vi "Skipfire.vi"(8 "error in (no error)":errorcluster, 11 "Node Ptr":T2 format="%.0x") -> (0 "error out":errorcluster)   [LabVIEW 2016, in "DCM System Explorer.lvlib"]
uses:
  DCM System Explorer.lvlib
  <vilib>/NI Veristand/Custom Device API/Custom Device Item Ref.ctl
  <vilib>/Powertrain Controls/Device Drivers/DCM/Skip Fire/RT/Skip Fire Setup.ctl
  Shared/DCM Properties.vi
  <vilib>/NI Veristand/Custom Device API/Get Item Property (String Array).vi
  Shared/DCM Constants and GUIDs.vi
  <vilib>/NI Veristand/Custom Device API/Set Item Property (String Array).vi
  <vilib>/NI VeriStand/Custom Device API/Custom Device API.lvlib
  DCM Shared.lvlib
  <vilib>/Powertrain Controls/Device Drivers/DCM/Skip Fire/RT/DCM - RT - Skip Fire.lvlib
panel:
  in  "_Setup Element":T1 caption="Command Setup"
  in  "_Refresh":bool
  in  "Channel Names":string[](array[string])=["", "", "", "", "", "", "", "", "", "", "", ""]
  in  "Channel Name":string
  in  "_Skipfire Channels":i32[](listbox) caption="Summary"
  in  "_Save Changes?":bool
  in  "Setup":T1[](array[typedef]) caption="Differential I/O Setup"
  in  "Header":cluster{"Section Name":string}={"Section Name"="Skip Fire Setup"}
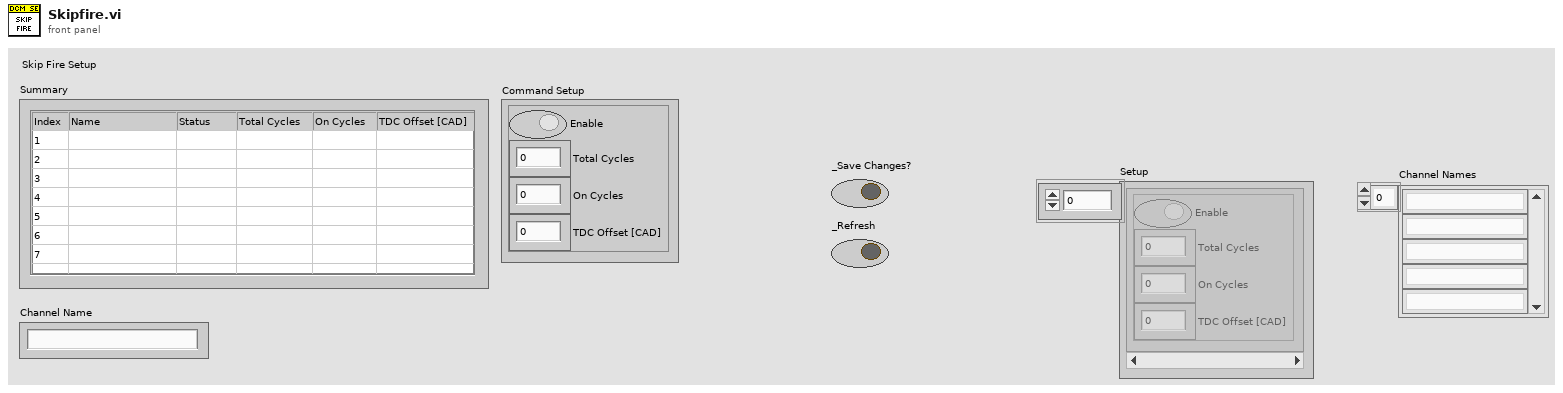
[diagram p1: front panel]
types:
  T1 = typedef "DCM - RT - Skip Fire.lvlib/Skip Fire Setup.ctl" = cluster{"Enable":bool, "Total Cycles":u8, "On Cycles":u8, "TDC Offset [CAD]":sgl}
  T2 = typedef "Custom Device API.lvlib/Custom Device Item Ref.ctl" = u64
  T3 = typedef "Custom Device API.lvlib/Custom Device Commands.ctl" = enum16{"Default", "Item renamed", "Shutdown", "Dynamic button pressed"}
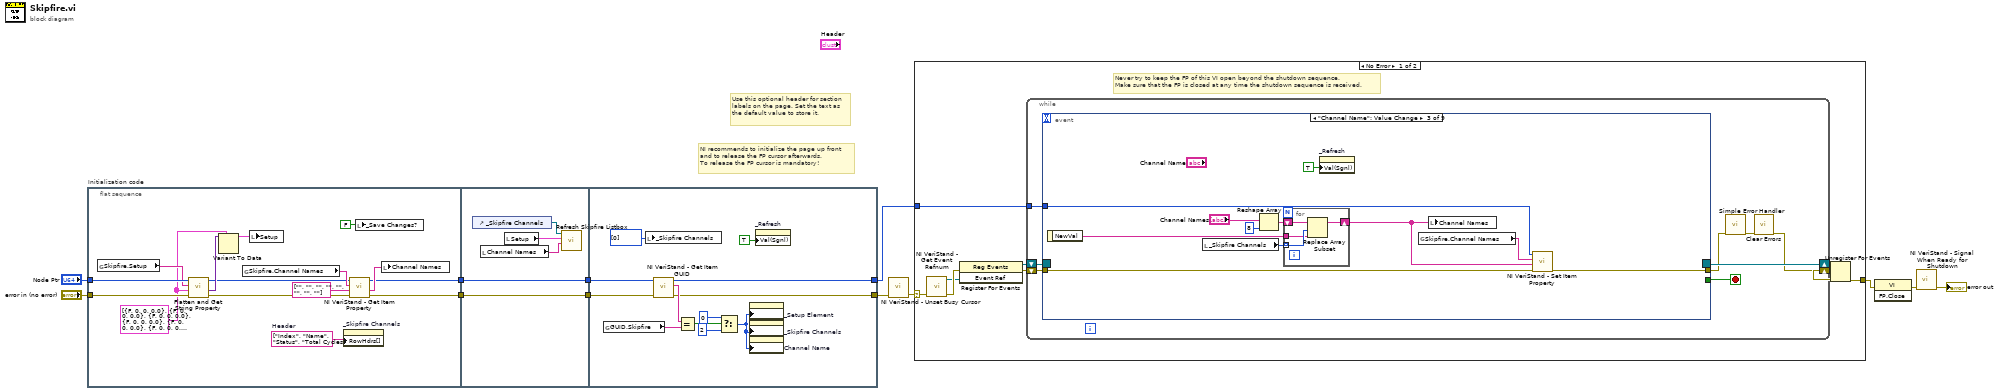
[diagram p0: block diagram]
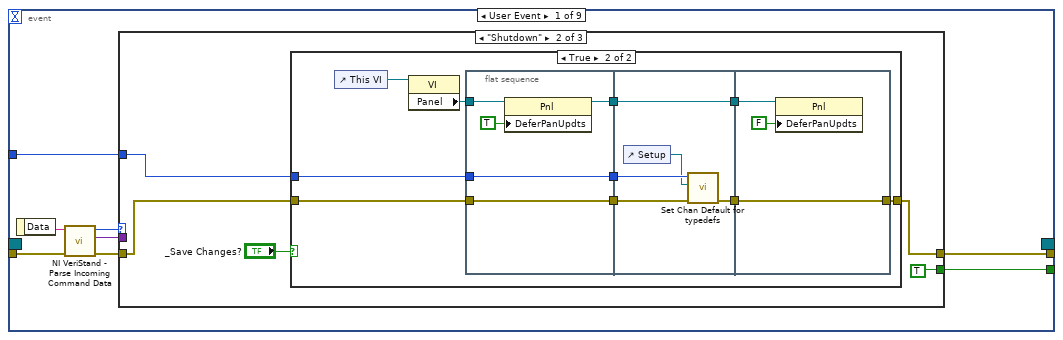
[diagram p2: hidden frame]
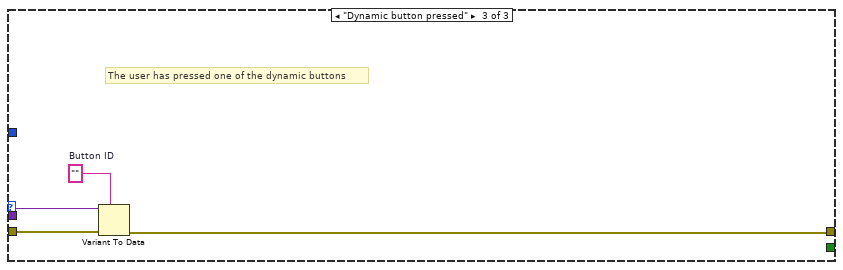
[diagram p5: hidden frame]
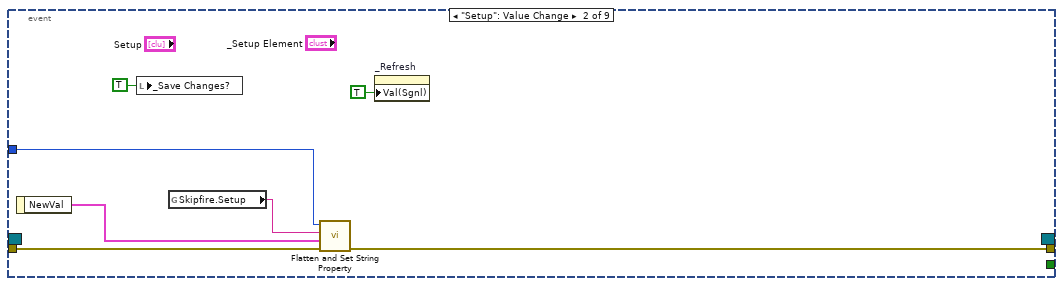
[diagram p6: hidden frame]
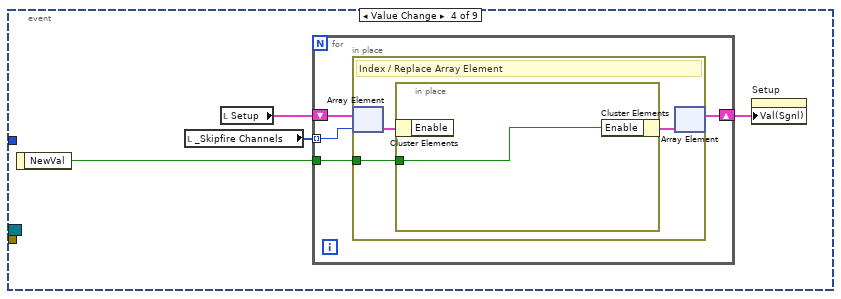
[diagram p7: hidden frame]
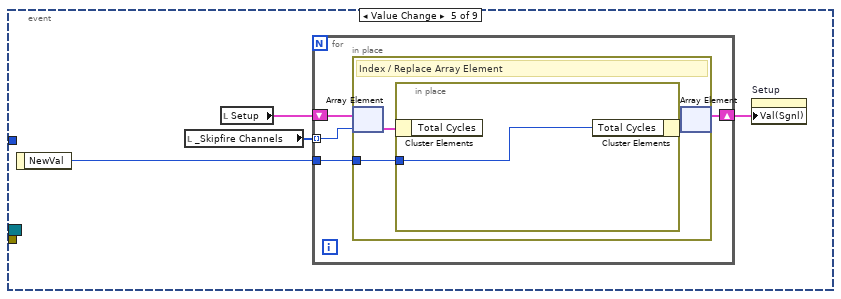
[diagram p8: hidden frame]
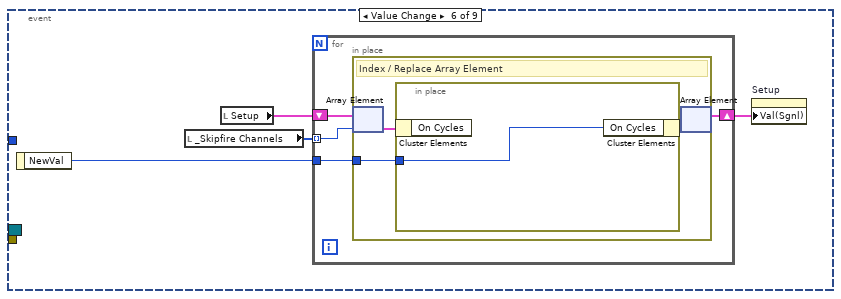
[diagram p9: hidden frame]
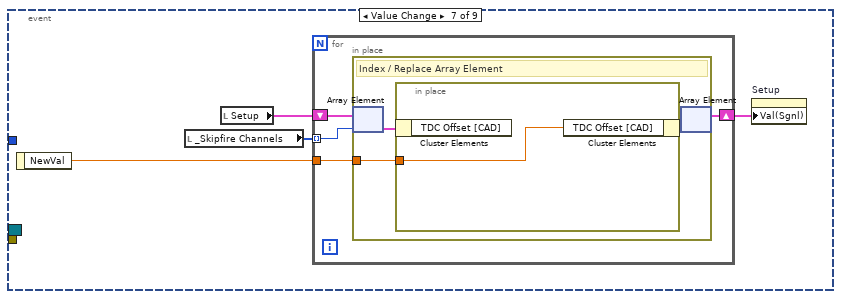
[diagram p10: hidden frame]
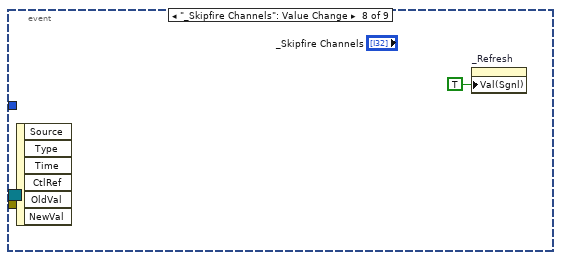
[diagram p11: hidden frame]
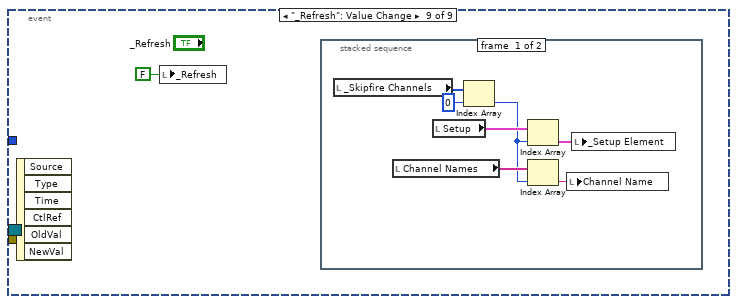
[diagram p12: hidden frame]
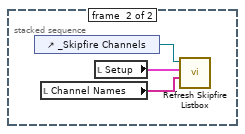
[diagram p13: hidden frame]
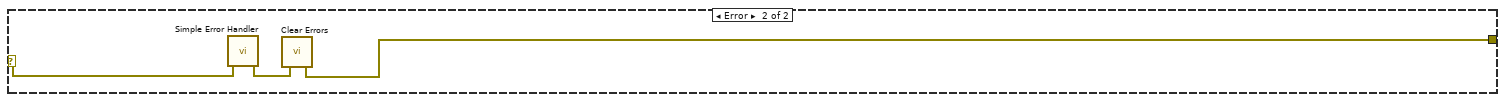
[diagram p14: hidden frame]
diagram:
  # "Use this optional header for section labels on the page. Set the text as the default value to store it."
  # "NI recommends to initialize the page up front\nand to release the FP cursor afterwards.\nTo release the FP cursor is mandatory!"
  n1 = flat-sequence "Initialization code" {
    tunnel: "Node Ptr" -> [w25]
    tunnel: "error in (no error)" -> [w26]
    tunnel: [w13] -> w5
    tunnel: [w14] -> w1
    tunnel: w5 -> [w31]
    tunnel: [w32] -> w4
    tunnel: [w31] -> w3
    tunnel: w1 -> [w32]
    tunnel: [w37] -> w2
    tunnel: [w36] -> w6
    tunnel: w4 -> [w39]
    tunnel: w3 -> [w38]
    frame #0 {
      w17 = string[] ["Index", "Name", "Status", "Total Cycles", "On Cycles", "TDC Offset [CAD]"]  # Header
      w23 = T1[] [{"Enable"=FALSE, "Total Cycles"=0, "On Cycles"=0, "TDC Offset [CAD]"=0.0}, {"Enable"=FALSE, "Total Cycles"=0, "On Cycles"=0, "TDC Offset [CAD]"=0.0}, {"Enable"=FALSE, "Total Cycles"=0, "On Cycles"=0, "TDC Offset [CAD]"=0.0}, {"Enable"=FALSE, "Total Cycles"=0, "On Cycles"=0, "TDC Offset [CAD]"=0.0}, {"Enable"=FALSE, "Total Cycles"=0, "On Cycles"=0, "TDC Offset [CAD]"=0.0}, {"Enable"=FALSE, "Total Cycles"=0, "On Cycles"=0, "TDC Offset [CAD]"=0.0}, {"Enable"=FALSE, "Total Cycles"=0, "On Cycles"=0, "TDC Offset [CAD]"=0.0}, {"Enable"=FALSE, "Total Cycles"=0, "On Cycles"=0, "TDC Offset [CAD]"=0.0}] ("DiffIO.Setup")
      n2 = global read "DCM Properties.vi" "Skipfire.Setup"() -> (w24:string)
      n3 = call "Flatten and Get String Property.vi"("error in (no error)"=w26, "Default Value"=w23, "Property Name"=w24, "Section Ref in"=w25) -> ("error out"=w15:errorcluster, "Value"=w27:variant, "Section Ref out"=w16:T2)  [unwired: 5 in]
      n4 = Variant To Data(type=w23, Variant=w27) -> (data=w22:T1[])  [unwired: 1 in, 1 out]
      n5 = global read "DCM Properties.vi" "Skipfire.Channel Names"() -> (w20:string)
      n6 = local write "Setup"(w22) -> ()
      n7 = property on="_Skipfire Channels" class="MCListbox (strict)"("RowHdrs[]"=w17) -> ()  [unwired: 2 in, 2 out]
      n8 = call-poly <vilib>:"NI VeriStand - Get Item Property.vi"("error in (no error)"=w15, "Default Value"=string[] ["", "", "", "", "", "", "", ""], "Property Name"=w20, "Item Ref in"=w16) -> ("error out"=w13:errorcluster, "Value"=w19:string[], "Item Ref out"=w14:T2)  [unwired: 4 in, 1 out]
      n9 = local write "_Save Changes?"(FALSE ("_Save Changes?")) -> ()
      n10 = local write "Channel Names"(w19) -> ()
    }
    frame #1 {
      n11 = control-ref of="_Skipfire Channels"() -> (w30:refnum<vi>)
      n12 = local read "Channel Names"() -> (w29:string[])
      n13 = local read "Setup"() -> (w28:T1[])
      n14 = call "Refresh Skipfire Listbox.vi"("ChannelNames"=w29, "Skipfire Settings Array"=w28, "Skipfire Listbox Refnum"=w30) -> ()  [unwired: 9 in]
    }
    frame #2 {
      n15 = global read "DCM Constants and GUIDs.vi" "GUID.Skipfire"() -> (w43:string)
      n16 = local write "_Skipfire Channels"(i32[] [0] ("_DiffIO Channels")) -> ()
      n17 = call <vilib>:"NI VeriStand - Get Item GUID.vi"("error in (no error)"=w38, "Item Ref in"=w39) -> ("error out"=w37:errorcluster, "GUID"=w42:string, "Item Ref out"=w36:T2)  [unwired: 7 in]
      n18 = Equal?(x=w42, y=w43) -> (x = y?=w44:bool)
      n19 = Select(t=0, s=w44, f=2) -> (s? t:f=w35:i32)
      n20 = property on="_Setup Element" class="Clust (strict)"("DisabledEnum"=w35) -> ()  [unwired: 2 in, 2 out]
      n21 = property on="_Skipfire Channels" class="MCListbox (strict)"("DisabledEnum"=w35) -> ()  [unwired: 2 in, 2 out]
      n22 = property on="Channel Name" class="Str"("DisabledEnum"=w35) -> ()  [unwired: 2 in, 2 out]
      n23 = property on="_Refresh" class="Bool (strict)"("Val(Sgnl)"=TRUE ("Value (Signaling)")) -> ()  [unwired: 2 in, 2 out]
    }
  }
  n24 = call <vilib>:"NI VeriStand - Unset Busy Cursor.vi"("error in (no error)"=w2) -> ("error out"=w8:errorcluster)  [unwired: 10 out]
  n25 = case shown="No Error" w8 {
    selector: w8 -> [w46 w188]
    tunnel: [w50 w186] -> w12
    tunnel: w6 -> [w45 _]
    frame No Error {
      # "Never try to keep the FP of this VI open beyond the shutdown sequence.\nMake sure that the FP is closed at any time the shutdown sequence is received."
      n26 = call <vilib>:"NI VeriStand - Get Event Refnum.vi"("error in (no error)"=w46) -> ("error out"=w53:errorcluster, "Event Ref"=w49:refnum<user-event>)  [unwired: 9 out]
      n27 = register-events(error in=w53, w49) -> (reference out=w47:refnum<event-registration>, error out=w48:errorcluster)  [unwired: 1 in]
      n28 = while {
        shift-right: [w55] -> w51
        shift-left: w48 -> [w60]
        shift-right: [w61] -> w52
        shift-left: w47 -> [w59]
        tunnel: w45 -> [w54]
        stop <- w58 stop-if-true
        n29 = event shown="[2] \"Channel Name\": Value Change" {
          selector: w59 -> [_ _ _ _ _ _ _ _ _]
          dyn-events: [_ _ _ _ _ _ _ _ _] -> w61
          timeout: _ -> [_ _ _ _ _ _ _ _ _]
          tunnel: w60 -> [w69 w110 w121 _ _ _ _ _ _]
          tunnel: [w65 _ _ _ _ _ _ _ _] -> w58
          tunnel: [w64 w109 w120 _ _ _ _ _ _] -> w57
          tunnel: w54 -> [w62 w106 w118 _ _ _ _ _ _]
          event User Event {
            n30 = event-data() -> ("Data"=w68:string)  [unwired: 1 out]
            n31 = call <vilib>:"NI VeriStand - Parse Incoming Command Data.vi"("error in (no error)"=w69, "Incoming data"=w68) -> ("error out"=w67:errorcluster, "Outgoing data"=w63:variant, "Action"=w66:T3)  [unwired: 7 out]
            n32 = case shown="\"Shutdown\"" w66 {
              tunnel: w67 -> [w70 w73 w103]
              tunnel: [_ TRUE _] -> w65
              tunnel: [w70 w72 w100] -> w64
              tunnel: w63 -> [_ _ w102]
              tunnel: w62 -> [_ w74 _]
              frame "Default", Default {
              }
              frame "Shutdown" {
                n33 = case shown="True" "_Save Changes?" {
                  tunnel: w74 -> [_ w81]
                  tunnel: w73 -> [w76 w80]
                  tunnel: [w76 w79] -> w72
                  frame False {
                  }
                  frame True {
                    n34 = control-ref of="This VI"() -> (w78:refnum<vi>)
                    n35 = property class="VI"(reference=w78) -> ("Panel"=w77:refnum<vi>)  [unwired: 1 in, 2 out]
                    n36 = flat-sequence {
                      tunnel: w80 -> [w90]
                      tunnel: w81 -> [w91]
                      tunnel: [w91] -> w86
                      tunnel: [w90] -> w85
                      tunnel: w77 -> [w89]
                      tunnel: [w87] -> w84
                      tunnel: w86 -> [w96]
                      tunnel: w85 -> [w95]
                      tunnel: [w94] -> w83
                      tunnel: [w93] -> w82
                      tunnel: w84 -> [w93]
                      tunnel: [w99] -> w79
                      tunnel: w83 -> [w99]
                      tunnel: w82 -> [w97]
                      frame #0 {
                        n37 = property class="Pnl"(reference=w89, "DeferPanUpdts"=TRUE ("Defer Panel Updates")) -> (reference out=w87:refnum<vi>)  [unwired: 1 in, 1 out]
                      }
                      frame #1 {
                        n38 = control-ref of="Setup"() -> (w92:refnum<vi>)
                        n39 = call "Set Chan Default for typedefs.vi"("error in"=w95, "Ctl Ref"=w92, "Section Ref in"=w96) -> ("error out"=w94:errorcluster)  [unwired: 7 in, 1 out]
                      }
                      frame #2 {
                        n40 = property class="Pnl"(reference=w97, "DeferPanUpdts"=FALSE ("Defer Panel Updates")) -> ()  [unwired: 1 in, 2 out]
                      }
                    }
                  }
                }
              }
              frame "Dynamic button pressed" {
                w101 = ""  # Button ID
                # "The user has pressed one of the dynamic buttons"
                n41 = Variant To Data(error in=w103, type=w101, Variant=w102) -> (error out=w100:errorcluster)  [unwired: 1 out]
              }
            }
          }
          event "Setup": Value Change {
            n42 = event-data() -> ("NewVal"=w107:T1[])  [unwired: 1 out]
            n43 = local write "_Save Changes?"(TRUE ("_Save Changes?")) -> ()
            n44 = global read "DCM Properties.vi" "Skipfire.Setup"() -> (w108:string)
            n45 = call "Flatten and Set String Property.vi"("error in (no error)"=w110, "Value"=w107, "Property Name"=w108, "Section Ref in"=w106) -> ("error out"=w109:errorcluster)  [unwired: 6 in, 1 out]
            n46 = property on="_Refresh" class="Bool (strict)"("Val(Sgnl)"=TRUE ("Value (Signaling)")) -> ()  [unwired: 2 in, 2 out]
          }
          event "Channel Name": Value Change {
            n47 = event-data() -> ("NewVal"=w114:string)  [unwired: 1 out]
            n48 = local read "_Skipfire Channels"() -> (w115:i32[])
            n49 = Reshape Array("Channel Names", 8 ("dimension size")) -> (w117:string[])
            n50 = for {
              tunnel: w115 -> [w123] mode=indexing
              shift-right: [w124] -> w111
              shift-left: w117 -> [w125]
              tunnel: w114 -> [w122]
              n51 = Replace Array Subset(array=w125, new element=w122, index=w123) -> (w124:string[])
            }
            n52 = property on="_Refresh" class="Bool (strict)"("Val(Sgnl)"=TRUE ("Value (Signaling)")) -> ()  [unwired: 2 in, 2 out]
            n53 = global read "DCM Properties.vi" "Skipfire.Channel Names"() -> (w119:string)
            n54 = local write "Channel Names"(w111) -> ()
            n55 = call-poly <vilib>:"NI VeriStand - Set Item Property.vi"("error in (no error)"=w121, "Value"=w111, "Property Name"=w119, "Item Ref in"=w118) -> ("error out"=w120:errorcluster)  [unwired: 5 in, 2 out]
          }
          event Value Change {
            n56 = event-data() -> ("NewVal"=w126:bool)  [unwired: 1 out]
            n57 = local read "_Skipfire Channels"() -> (w127:i32[])
            n58 = local read "Setup"() -> (w128:T1[])
            n59 = for {
              tunnel: w127 -> [w132] mode=indexing
              shift-right: [w131] -> w129
              shift-left: w128 -> [w133]
              tunnel: w126 -> [w130]
              n60 = in-place {
                in-place-border: w130 -> [w134]
                # "Index / Replace Array Element"
                n61 = in-place-array #1(w133, w132) -> (w136:T1)
                n62 = in-place {
                  in-place-border: w134 -> [w137]
                  n63 = in-place-cluster #2(w136) -> ()  [unwired: 1 out]
                  n64 = in-place-cluster #2("Enable"=w137) -> (w135:T1)
                }
                n65 = in-place-array #1(w135) -> (w131:T1[])  [unwired: 1 out]
              }
            }
            n66 = property on="Setup" class="Arr (strict)"("Val(Sgnl)"=w129) -> ()  [unwired: 2 in, 2 out]
          }
          event Value Change {
            n67 = event-data() -> ("NewVal"=w138:u8)  [unwired: 1 out]
            n68 = local read "_Skipfire Channels"() -> (w139:i32[])
            n69 = local read "Setup"() -> (w140:T1[])
            n70 = for {
              tunnel: w139 -> [w144] mode=indexing
              shift-right: [w143] -> w141
              shift-left: w140 -> [w145]
              tunnel: w138 -> [w142]
              n71 = in-place {
                in-place-border: w142 -> [w146]
                # "Index / Replace Array Element"
                n72 = in-place-array #3(w145, w144) -> (w148:T1)
                n73 = in-place {
                  in-place-border: w146 -> [w149]
                  n74 = in-place-cluster #4(w148) -> ()  [unwired: 1 out]
                  n75 = in-place-cluster #4("Total Cycles"=w149) -> (w147:T1)
                }
                n76 = in-place-array #3(w147) -> (w143:T1[])  [unwired: 1 out]
              }
            }
            n77 = property on="Setup" class="Arr (strict)"("Val(Sgnl)"=w141) -> ()  [unwired: 2 in, 2 out]
          }
          event Value Change {
            n78 = event-data() -> ("NewVal"=w150:u8)  [unwired: 1 out]
            n79 = local read "_Skipfire Channels"() -> (w151:i32[])
            n80 = local read "Setup"() -> (w152:T1[])
            n81 = for {
              tunnel: w151 -> [w156] mode=indexing
              shift-right: [w155] -> w153
              shift-left: w152 -> [w157]
              tunnel: w150 -> [w154]
              n82 = in-place {
                in-place-border: w154 -> [w158]
                # "Index / Replace Array Element"
                n83 = in-place-array #5(w157, w156) -> (w160:T1)
                n84 = in-place {
                  in-place-border: w158 -> [w161]
                  n85 = in-place-cluster #6(w160) -> ()  [unwired: 1 out]
                  n86 = in-place-cluster #6("On Cycles"=w161) -> (w159:T1)
                }
                n87 = in-place-array #5(w159) -> (w155:T1[])  [unwired: 1 out]
              }
            }
            n88 = property on="Setup" class="Arr (strict)"("Val(Sgnl)"=w153) -> ()  [unwired: 2 in, 2 out]
          }
          event Value Change {
            n89 = event-data() -> ("NewVal"=w162:sgl)  [unwired: 1 out]
            n90 = local read "_Skipfire Channels"() -> (w163:i32[])
            n91 = local read "Setup"() -> (w164:T1[])
            n92 = for {
              tunnel: w163 -> [w168] mode=indexing
              shift-right: [w167] -> w165
              shift-left: w164 -> [w169]
              tunnel: w162 -> [w166]
              n93 = in-place {
                in-place-border: w166 -> [w170]
                # "Index / Replace Array Element"
                n94 = in-place-array #7(w169, w168) -> (w172:T1)
                n95 = in-place {
                  in-place-border: w170 -> [w173]
                  n96 = in-place-cluster #8(w172) -> ()  [unwired: 1 out]
                  n97 = in-place-cluster #8("TDC Offset [CAD]"=w173) -> (w171:T1)
                }
                n98 = in-place-array #7(w171) -> (w167:T1[])  [unwired: 1 out]
              }
            }
            n99 = property on="Setup" class="Arr (strict)"("Val(Sgnl)"=w165) -> ()  [unwired: 2 in, 2 out]
          }
          event "_Skipfire Channels": Value Change {
            n100 = event-data() -> ()  [unwired: 7 out]
            n101 = property on="_Refresh" class="Bool (strict)"("Val(Sgnl)"=TRUE ("Value (Signaling)")) -> ()  [unwired: 2 in, 2 out]
          }
          event "_Refresh": Value Change {
            n102 = event-data() -> ()  [unwired: 7 out]
            n103 = local write "_Refresh"(FALSE ("_Refresh")) -> ()
            n104 = stacked-sequence {
              frame #0 {
                n105 = local read "_Skipfire Channels"() -> (w178:i32[])
                n106 = local read "Channel Names"() -> (w182:string[])
                n107 = local read "Setup"() -> (w180:T1[])
                n108 = Index Array(array=w178, index=0) -> (element=w177:i32)
                n109 = Index Array(array=w180, index=w177) -> (element=w179:T1)
                n110 = Index Array(array=w182, index=w177) -> (element=w181:string)
                n111 = local write "Channel Name"(w181) -> ()
                n112 = local write "_Setup Element"(w179) -> ()
              }
              frame #1 {
                n113 = control-ref of="_Skipfire Channels"() -> (w184:refnum<vi>)
                n114 = local read "Channel Names"() -> (w183:string[])
                n115 = local read "Setup"() -> (w185:T1[])
                n116 = call "Refresh Skipfire Listbox.vi"("ChannelNames"=w183, "Skipfire Settings Array"=w185, "Skipfire Listbox Refnum"=w184) -> ()  [unwired: 9 in]
              }
            }
          }
        }
        n117 = call <vilib>:"Simple Error Handler.vi"("error in (no error)"=w57) -> ("error out"=w56:errorcluster)  [unwired: 1 in, 7 out]
        n118 = call <vilib>:"Clear Errors.vi"("error in (no error)"=w56) -> ("error out"=w55:errorcluster)  [unwired: 1 in, 5 out]
      }
      n119 = Unregister For Events(event registration refnum=w52, error in=w51) -> (error out=w50:errorcluster)
    }
    frame Error {
      n120 = call <vilib>:"Simple Error Handler.vi"("error in (no error)"=w188) -> ("error out"=w187:errorcluster)  [unwired: 1 in, 7 out]
      n121 = call <vilib>:"Clear Errors.vi"("error in (no error)"=w187) -> ("error out"=w186:errorcluster)  [unwired: 1 in, 5 out]
    }
  }
  n122 = invoke class="VI" method="FP.Close"(error in=w12) -> (error out=w11:errorcluster)  [unwired: 2 in, 2 out]
  n123 = call <vilib>:"NI VeriStand - Signal When Ready for Shutdown.vi"("error in (no error)"=w11) -> ("error out"=→"error out":errorcluster)  [unwired: 10 out]
